vi "Set RPC ConfigureDMM __Output.vi"(7 "Streeming? (F)":bool, 8 "error in (no error)":errorcluster, 10 "Message Data":T1, 11 "gRPCid in":T3) -> (0 "error out":errorcluster)   [LabVIEW 2019, in "HVC3.lvlib" / "HVC3.lvclass"]
uses:
  HVC3.lvclass
  gRPC lvSupport/Server API/typeDefs/grpcId.ctl
  RPC Messages/measurementservice_DMMConfigResponse/measurementservice_DMMConfigResponse_Data.ctl
  RPC Messages/measurementservice_ErrorOut/measurementservice_ErrorOut_Data.ctl
  gRPC lvSupport/gprc-lvsupport.lvlib
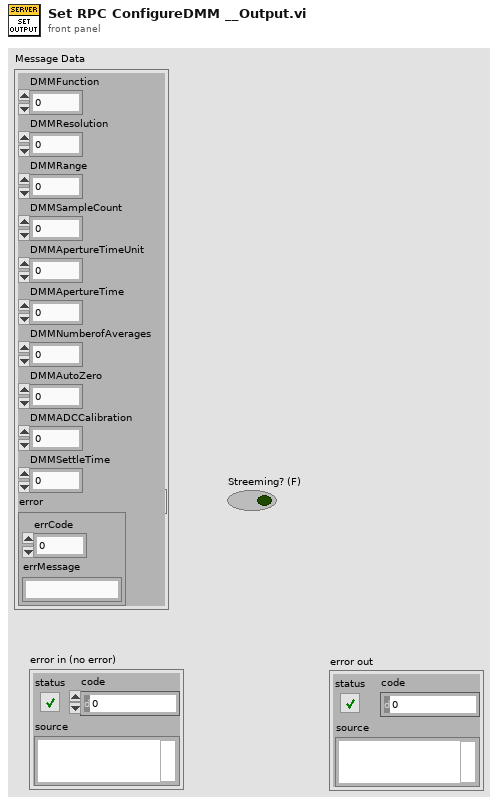
[diagram p1: front panel]
types:
  T1 = typedef "HVC3.lvlib/HVC3.lvclass/measurementservice_DMMConfigResponse_Data.ctl" = cluster{"DMMFunction":i32, "DMMResolution":sgl, "DMMRange":sgl, "DMMSampleCount":i32, "DMMApertureTimeUnit":i32, "DMMApertureTime":sgl, "DMMNumberofAverages":i32, "DMMAutoZero":i32, "DMMADCCalibration":i32, "DMMSettleTime":sgl, "error":T2}
  T2 = typedef "HVC3.lvlib/HVC3.lvclass/measurementservice_ErrorOut_Data.ctl" = cluster{"errCode":i32, "errMessage":string}
  T3 = typedef "HVC3.lvlib/gprc-lvsupport.lvlib/grpcId.ctl" = u64
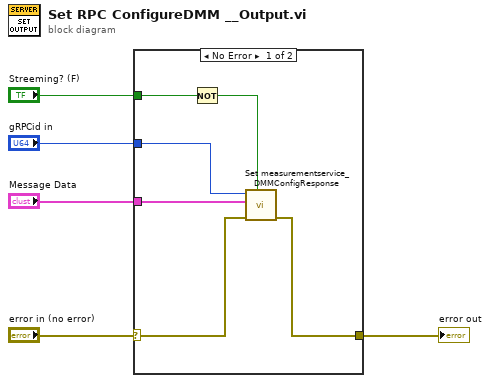
[diagram p0: block diagram]
diagram:
  n1 = case shown="No Error" "error in (no error)" {
    selector: "error in (no error)" -> [w11 w12]
    tunnel: [w9 w12] -> w4
    tunnel: "gRPCid in" -> [w10 _]
    tunnel: "Message Data" -> [w8 _]
    tunnel: "Streeming? (F)" -> [w7 _]
    frame No Error {
      n2 = Not(x=w7) -> (.not. x?=w6:bool)
      n3 = call "Set measurementservice_DMMConfigResponse.vi"("Complete Call (T)"=w6, "error in (no error)"=w11, "Message Data"=w8, "gRPCid"=w10) -> ("error out"=w9:errorcluster)  [unwired: 7 in]
    }
    frame Error {
    }
  }
  "error out" <- w4
